vi "Actor Core.vi"(8 "error in":errorcluster, 11 "Chat Room Model in":refnum<class "Chat Window Model.lvclass">) -> (0 "error out":errorcluster, 3 "Actor out":refnum<class "Actor.lvclass">)   [LabVIEW 2020, in "Chat Room Model.lvlib" / "Chat Window Model.lvclass"]
doc: "(<B>Filename</B>: Actor Framework.lvlib:Actor.lvclass:Actor Core.vi)\n\nReceives messages to the actor, reacts to them, and initiates any error handling that may shut the actor down.\n\nDescendant classes may override this VI to append parallel tasks for the actor to complete while it handles messages. Overrides use the Call Parent Class Method node."
uses:
  Chat Window Model.lvclass
  C:/Program Files (x86)/National Instruments/LabVIEW 2020/vi.lib/ActorFramework/Actor/Actor.lvclass
  <vilib>/ActorFramework/Actor/Actor.lvclass
  Chat Window UI/Chat Window Controller UI.lvclass
  F:/Gitlab Repository/LabVIEW-Study/10.Top 5 Actor Framework Overrides/Chat Room with Interface/Chat Window UI Controller/Chat Window UI Controller/Chat Window Controller.lvclass
  Chat Window Model.lvclass/Chat Window Model.ctl
  Chat Window UI Controller/Chat Window UI Controller/Chat Window Controller.lvclass/Chat Window Controller.ctl
  Chat Window UI Controller/Chat Window UI Controller/Chat Window Controller.lvclass
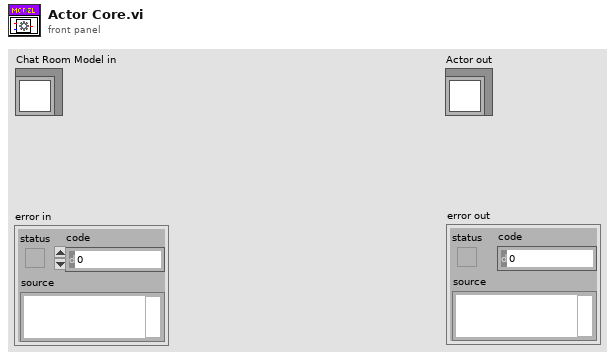
[diagram p1: front panel]
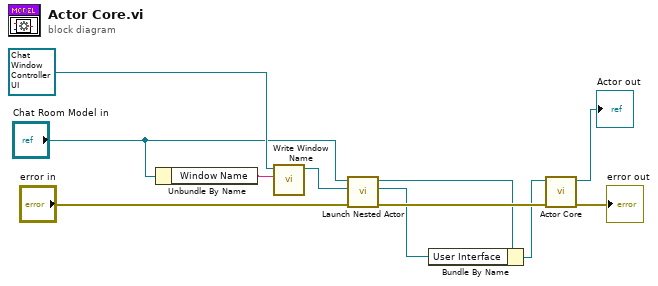
[diagram p0: block diagram]
diagram:
  n1 = Unbundle By Name("Chat Room Model in") -> ("Window Name"=w1:string)
  n2 = call "Write Window Name.vi"("Window Name"=w1, "Chat Window Controller in"=refnum<class "Chat Window Controller UI.lvclass"> refnum ("Chat Window UI.lvlib:Chat Window UI.lvclass")) -> ("Chat Window Controller out"=w3:refnum<class "Chat Window Controller UI.lvclass">)  [unwired: 8 in, 1 out]
  n3 = call <vilib>:"Launch Nested Actor.vi"("error in (no error)"="error in", "Nested Actor"=w3, "Caller Actor in"="Chat Room Model in") -> ("error out"=w9:errorcluster, "Nested Actor's Enqueuer"=w6:refnum<class "Message Enqueuer.lvclass">, "Caller Actor out"=w7:refnum<class "Chat Window Model.lvclass">)  [unwired: 6 in]
  n4 = Bundle By Name(cluster=w7, "User Interface"=w6) -> (w5:refnum<class "Chat Window Model.lvclass">)
  n5 = call-parent "Actor Core.vi"("error in"=w9, "Actor in"=w5) -> ("error out"=→"error out":errorcluster, "Actor out"=→"Actor out":refnum<class "Actor.lvclass">)  [unwired: 8 in]
